vi "send data.vi"(11 "Template in":refnum<class "Template.lvclass">) -> (0 "error out":errorcluster)   [LabVIEW 2020, in "Template.lvlib" / "Template.lvclass"]
doc: "Dequeues the local actor DVR and sends this DVR to the Pool registered by the root actor, where it will be read and acted upon"
uses:
  Template.lvclass
  Template.lvclass/Template.ctl
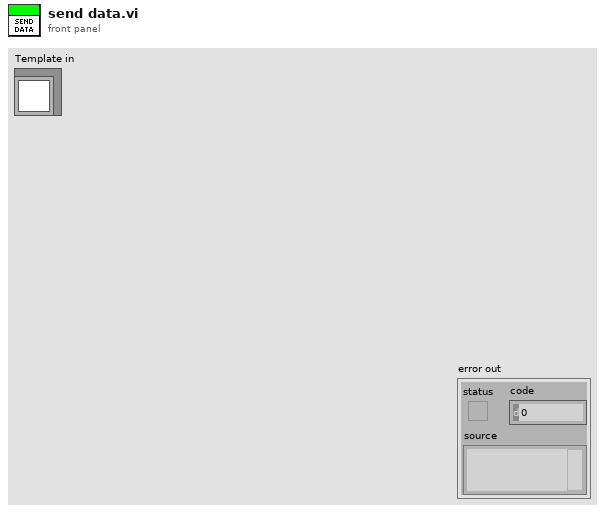
[diagram p1: front panel]
types:
  T1 = typedef "Template.lvlib/Template.lvclass/base actor notifiers.ctl" = cluster{"Stop Actor":refnum<notifier>, "UI Data":refnum<notifier>}
  T2 = typedef "Template.lvlib/Template.lvclass/base actor queues.ctl" = cluster{"DVR Pool":refnum<queue>, "Actor's Data":refnum<queue>}
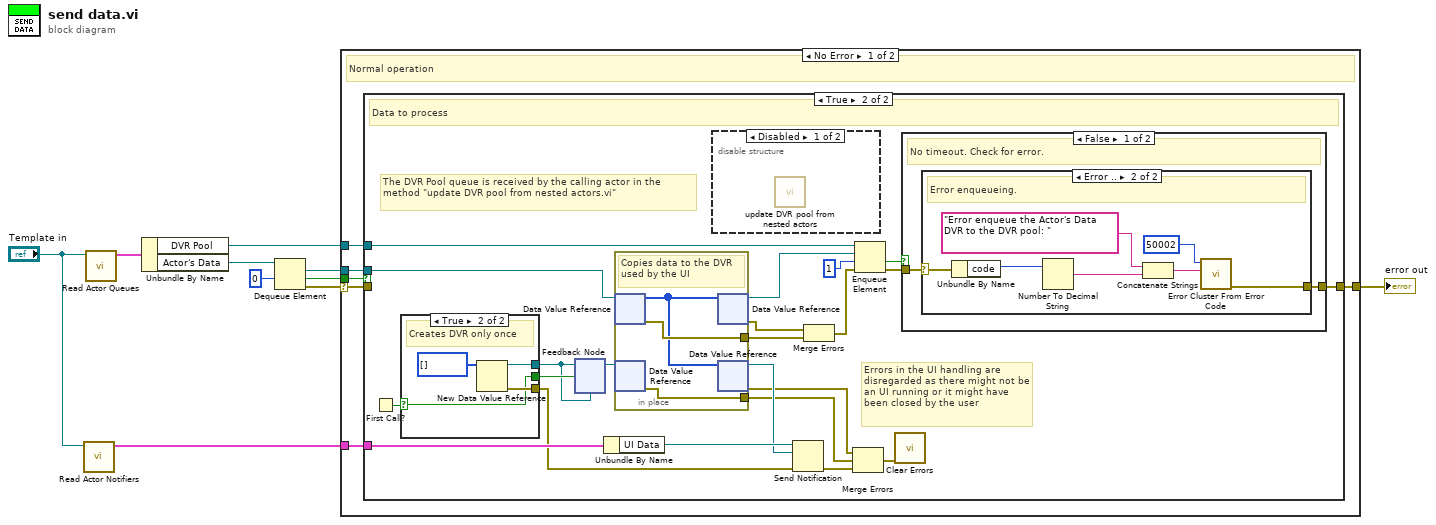
[diagram p0: block diagram]
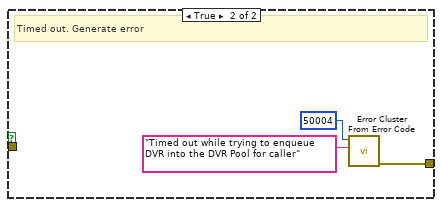
[diagram p6: hidden frame]
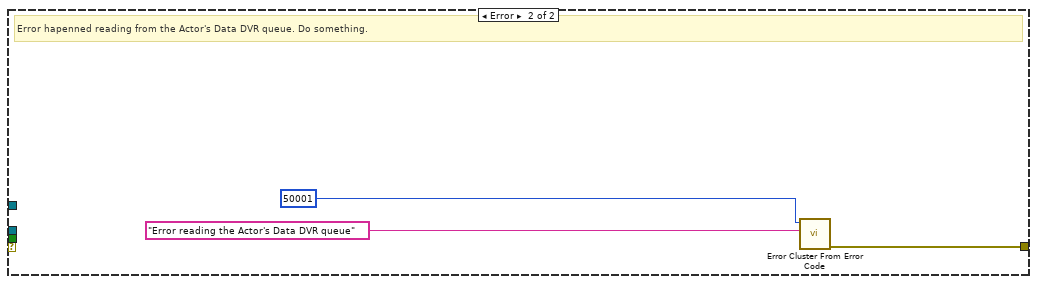
[diagram p7: hidden frame]
diagram:
  n1 = call "Read Actor Notifiers.vi"("Template in"="Template in") -> ("Base Actor Notifiers"=w1:T1)  [unwired: 10 in]
  n2 = call "Read Actor Queues.vi"("Template in"="Template in") -> ("Base Actor Queues"=w10:T2)  [unwired: 10 in]
  n3 = Unbundle By Name(w10) -> ("DVR Pool"=w8:refnum<queue>, "Actor's Data"=w7:refnum<queue>)
  n4 = Dequeue Element(queue=w7, timeout in ms (-1)=0) -> (element=w6:refnum<data-value>, timed out?=w4:bool, error out=w3:errorcluster)  [unwired: 1 in, 1 out]
  n5 = case shown="No Error" w3 {
    selector: w3 -> [w12 _]
    tunnel: [w16 w62] -> w9
    tunnel: w8 -> [w15 _]
    tunnel: w6 -> [w14 _]
    tunnel: w4 -> [w13 _]
    tunnel: w1 -> [w11 _]
    frame No Error {
      # "Normal operation"
      n6 = case shown="True" w13 {
        tunnel: [w17 w36] -> w16
        tunnel: w15 -> [_ w39]
        tunnel: w14 -> [_ w34]
        tunnel: w12 -> [w17 _]
        tunnel: w11 -> [_ w29]
        frame False {
          # "No Data to Process"
        }
        frame True {
          # "The DVR Pool queue is received by the calling actor in the method \"update DVR pool from nested actors.vi\""
          # "Errors in the UI handling are disregarded as there might not be an UI running or it might have been closed by the user"
          # "Data to process"
          n7 = First Call?() -> (First Call?: T/F=w27:bool)
          n8 = case shown="True" w27 {
            selector: w27 -> [w40 w41]
            tunnel: [_ w43] -> w24
            tunnel: [_ w42] -> w22
            tunnel: [w40 w41] -> w25
            frame False {
              # "Uses same DVR"
            }
            frame True {
              # "Creates DVR only once"
              n9 = New Data Value Reference(data value=u8[] []) -> (data value reference=w43:refnum<data-value>, error out=w42:errorcluster)  [unwired: 1 in]
            }
          }
          n10 = feedback #1(w24) -> (w26:refnum<data-value>)
          n11 = feedback-in #1(w24, w25) -> ()
          n12 = Unbundle By Name(w29) -> ("UI Data"=w28:refnum<notifier>)
          n13 = in-place {
            in-place-border: [w47] -> w32
            in-place-border: [w45] -> w20
            # "Copies data to the DVR used by the UI"
            n14 = in-place-dvr #2(w34) -> (w46:u8[], w47:errorcluster)
            n15 = in-place-dvr #3(w26) -> (w45:errorcluster)  [unwired: 1 out]
            n16 = in-place-dvr #2(w46) -> (w33:refnum<data-value>, w30:errorcluster)
            n17 = in-place-dvr #3(w46) -> (w23:refnum<data-value>, w19:errorcluster)
          }
          n18 = disable-structure shown="Disabled" {
            frame Disabled {
              n19 = call "update DVR pool from nested actors.vi"() -> ()  [unwired: 11 in, 1 out]
            }
            frame Enabled {
            }
          }
          n20 = Send Notification(notification=w23, notifier=w28, error in (no error)=w22) -> (error out=w21:errorcluster)  [unwired: 1 out]
          n21 = Merge Errors(w30, w32) -> (w31:errorcluster)
          n22 = Merge Errors(w19, w20, w21) -> (w18:errorcluster)
          n23 = Enqueue Element(queue=w39, element=w33, timeout in ms (-1)=1, error in (no error)=w31) -> (timed out?=w35:bool, error out=w37:errorcluster)  [unwired: 1 out]
          n24 = call <vilib>:"Clear Errors.vi"("error in (no error)"=w18) -> ()  [unwired: 5 in, 2 out]
          n25 = case shown="False" w35 {
            tunnel: w37 -> [w49 _]
            tunnel: [w48 w59] -> w36
            frame False {
              # "No timeout. Check for error."
              n26 = case shown="Error .." w49 {
                selector: w49 -> [_ w53]
                tunnel: [_ w54] -> w48
                frame No Error {
                  # "Normal operation"
                }
                frame Error {
                  # "Error enqueueing."
                  n27 = Unbundle By Name(w53) -> ("code"=w52:i32)
                  n28 = Number To Decimal String(number=w52) -> (decimal integer string=w50:string)  [unwired: 1 in]
                  n29 = Concatenate Strings("Error enqueue the Actor's Data DVR to the DVR pool: " ("error message (\"\")"), w50) -> (w51:string)
                  n30 = call <vilib>:"Error Cluster From Error Code.vi"("error message (\"\")"=w51, "error code (0)"=50002) -> ("error out"=w54:errorcluster)  [unwired: 7 in]
                }
              }
            }
            frame True {
              # "Timed out. Generate error"
              n31 = call <vilib>:"Error Cluster From Error Code.vi"("error message (\"\")"="Timed out while trying to enqueue DVR into the DVR Pool for caller" ("error message (\"\")"), "error code (0)"=50004) -> ("error out"=w59:errorcluster)  [unwired: 7 in]
            }
          }
        }
      }
    }
    frame Error {
      # "Error hapenned reading from the Actor's Data DVR queue. Do something."
      n32 = call <vilib>:"Error Cluster From Error Code.vi"("error message (\"\")"="Error reading the Actor's Data DVR queue" ("error message (\"\")"), "error code (0)"=50001) -> ("error out"=w62:errorcluster)  [unwired: 7 in]
    }
  }
  "error out" <- w9
